vi "Read Model case running.vi"(8 "error in (no error)":errorcluster, 11 "Fiber Auto Collimation state data in":refnum<class "Fiber Auto Collimation state data.lvclass">) -> (0 "error out":errorcluster, 1 "Model is idle":bool, 2 "Model case running":string, 3 "Fiber Auto Collimation state data out":refnum<class "Fiber Auto Collimation state data.lvclass">, 4 "Enabled only if idle":T1(ring))   [LabVIEW 2018, in "Fiber Auto Collimation state data.lvclass"]
doc: "This is the current state running on the main Model loop. If nothing is running, then this is \"Idle\".\n\nThere is an output added to make it easier to enable controls only when the model is idle, which is a pretty common thing to do in the View loop."
uses:
  Fiber Auto Collimation state data.lvclass
  Fiber Auto Collimation state data.lvclass/Fiber Auto Collimation state data.ctl
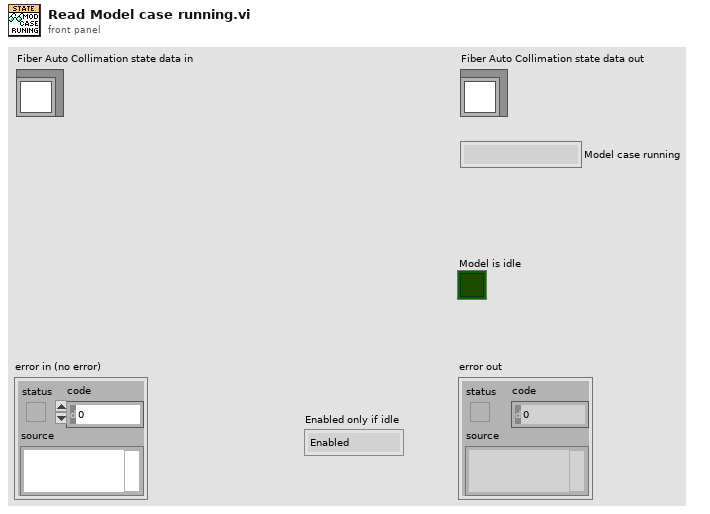
[diagram p1: front panel]
types:
  T1 = enum8{"Enabled", "Disabled", "Disabled and Grayed Out"}
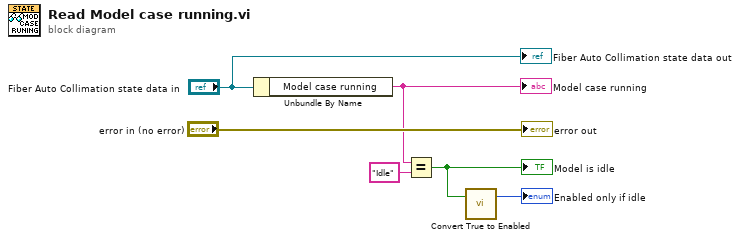
[diagram p0: block diagram]
diagram:
  n1 = Unbundle By Name("Fiber Auto Collimation state data in") -> ("Model case running"=w4:string)
  "Model case running" <- w4
  n2 = Equal?(x=w4, y="Idle") -> (x = y?=w2:bool)
  "Model is idle" <- w2
  n3 = call <userlib>:"Convert True to Enabled.vi"("Enable?"=w2) -> ("Enabled"=→"Enabled only if idle":T1)  [unwired: 2 in]
  "error out" <- "error in (no error)"
  "Fiber Auto Collimation state data out" <- "Fiber Auto Collimation state data in"
